vi "Read Self-Test Result Message.vi"(8 "error in (no error)":errorcluster, 11 "CSPP_DeviceGUIActor":refnum<class "CSPP_DeviceGUIActor.lvclass">) -> (0 "error out":errorcluster, 2 "Self-Test Result Message":string, 3 "CSPP_DeviceGUIActor":refnum<class "CSPP_DeviceGUIActor.lvclass">)   [LabVIEW 2016, in "CSPP_DeviceGUIActor.lvlib" / "CSPP_DeviceGUIActor.lvclass"]
doc: "Returns the self-test response string from the instrument. See the instrument's operation manual for an explanation of the string's contents.\n\nThis value has been read at launch time of actor once."
uses:
  CSPP_DeviceGUIActor.lvclass
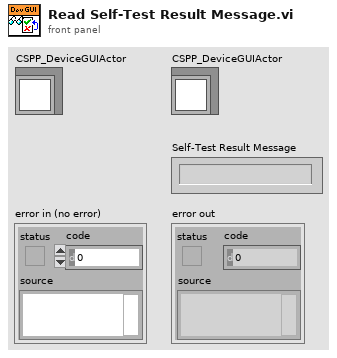
[diagram p1: front panel]
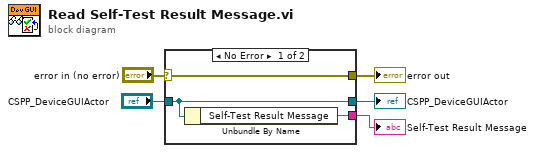
[diagram p0: block diagram]
diagram:
  n1 = case shown="No Error" "error in (no error)" {
    selector: "error in (no error)" -> [w8 w9]
    tunnel: [w8 w9] -> w4
    tunnel: [w7 w10] -> w2
    tunnel: "CSPP_DeviceGUIActor" -> [w7 w10]
    tunnel: [w6 _] -> w1
    frame No Error {
      n2 = Unbundle By Name(w7) -> ("Self-Test Result Message"=w6:string)
    }
    frame Error {
    }
  }
  "error out" <- w4
  "CSPP_DeviceGUIActor" <- w2
  "Self-Test Result Message" <- w1
